vi "(SubVI) number_SET_rule_in_12_cards.vi"(1 "array_ID":dbl[](array[numeric])) -> (0 "Matching_idx":i32[][](array[numeric]))   [LabVIEW 2018]
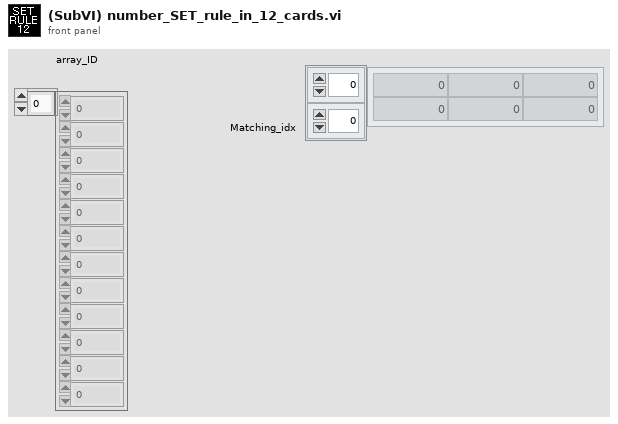
[diagram p1: front panel]
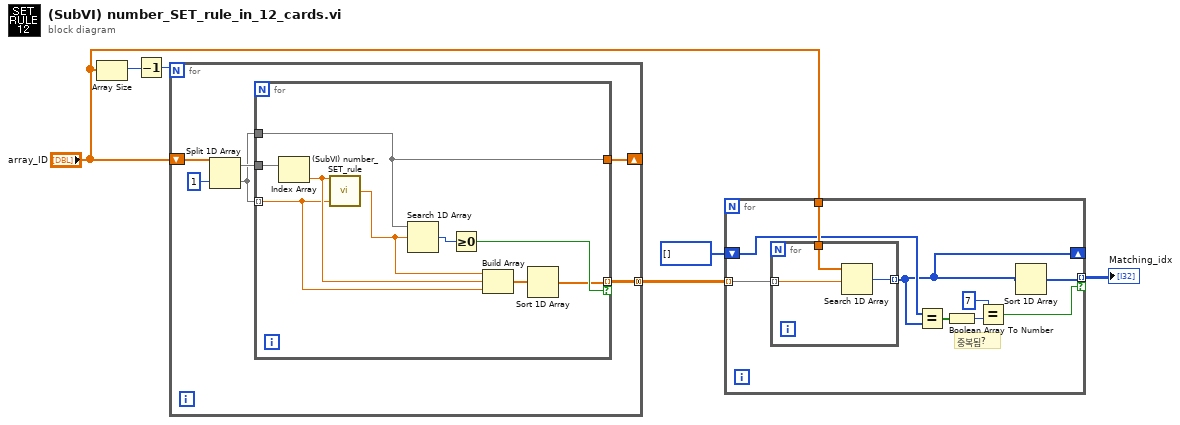
[diagram p0: block diagram]
diagram:
  n1 = Array Size(array="array_ID") -> (size(s)=w5:i32)
  n2 = Decrement(x=w5) -> (x-1=w6:i32)
  n3 = for {
    N: w6 -> [_]
    shift-right: [w8] -> _
    shift-left: "array_ID" -> [w11]
    tunnel: [w7] -> w4 mode=concatenating
    n4 = Split 1D Array(array=w11, index=1 ("인덱스")) -> (first subarray=w10:dbl[], second subarray=w9:dbl[])
    n5 = for {
      tunnel: w10 -> [w21]
      tunnel: w9 -> [w16] mode=indexing
      tunnel: w9 -> [w19]
      tunnel: [w19] -> w8
      tunnel: [w13] -> w7 mode=indexing if=w15
      n6 = Index Array(array=w21) -> (element=w17:dbl)  [unwired: 1 in]
      n7 = call "(SubVI) number_SET_rule.vi"("Input_2"=w16, "Input_1"=w17) -> ("Matching_number"=w18:dbl)
      n8 = Search 1D Array(1D array=w19, element=w18) -> (index of element=w20:i32)  [unwired: 1 in]
      n9 = Greater Or Equal To 0?(x=w20) -> (x >= 0?=w15:bool)
      n10 = Build Array(w18, w17, w16) -> (w14:dbl[])
      n11 = Sort 1D Array(array=w14) -> (sorted array=w13:dbl[])
    }
  }
  n12 = for {
    tunnel: w4 -> [w29] mode=indexing
    tunnel: "array_ID" -> [w30]
    shift-right: [w23] -> _
    shift-left: i32[] [] ("Matching_idx 2") -> [w28]
    tunnel: [w22] -> w1 mode=indexing if=w24
    # "중복됨?"
    n13 = for {
      tunnel: w30 -> [w33]
      tunnel: w29 -> [w32] mode=indexing
      tunnel: [w31] -> w23 mode=indexing
      n14 = Search 1D Array(1D array=w33, element=w32) -> (index of element=w31:i32)  [unwired: 1 in]
    }
    n15 = Equal?(x=w28, y=w23) -> (x = y?=w27:bool[])
    n16 = Boolean Array To Number(Boolean array=w27) -> (number=w26:u32)
    n17 = Equal?(x=u32 7, y=w26) -> (x = y?=w24:bool)
    n18 = Sort 1D Array(array=w23) -> (sorted array=w22:i32[])
  }
  "Matching_idx" <- w1
